vi "Win Host - Decimate Image Low Level.vi"(8 "error in (no error)":errorcluster, 11 "Image Path":path) -> (0 "error out":errorcluster, 1 "ImageData":T1, 2 "Rectangle":T2, 3 "new picture":picture)   [LabVIEW 2024]
uses:
  <vilib>/picture/picture.llb/imagedata.ctl
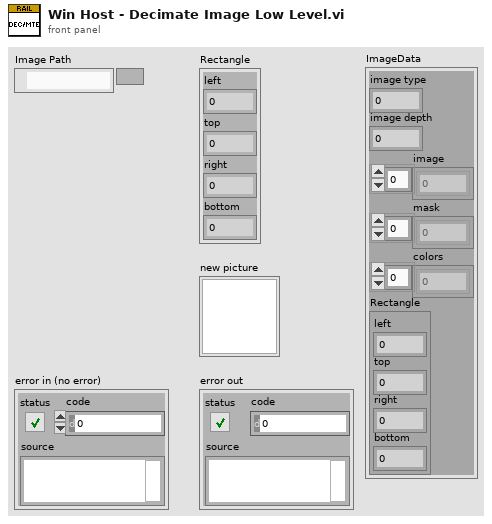
[diagram p1: front panel]
types:
  T1 = typedef "imagedata.ctl" = cluster{"image type":i32, "image depth":i32, "image":u8[], "mask":u8[], "colors":u32[], "Rectangle":cluster{"left":i16, "top":i16, "right":i16, "bottom":i16}}
  T2 = cluster{"left":i16, "top":i16, "right":i16, "bottom":i16}
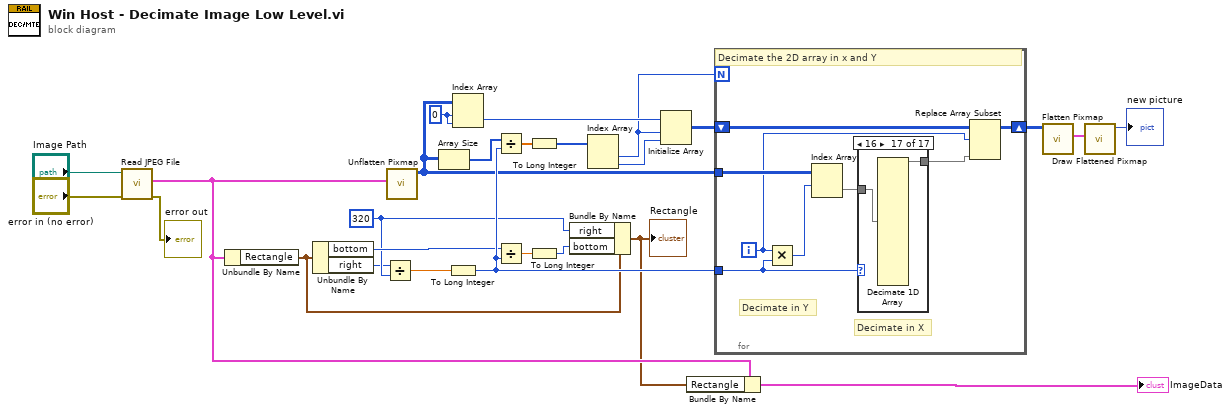
[diagram p0: block diagram]
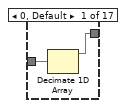
[diagram p2: hidden frame]
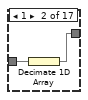
[diagram p3: hidden frame]
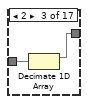
[diagram p4: hidden frame]
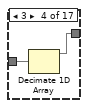
[diagram p5: hidden frame]
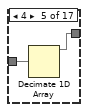
[diagram p6: hidden frame]
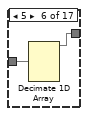
[diagram p7: hidden frame]
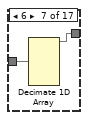
[diagram p8: hidden frame]
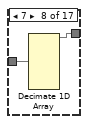
[diagram p9: hidden frame]
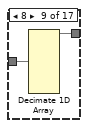
[diagram p10: hidden frame]
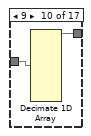
[diagram p11: hidden frame]
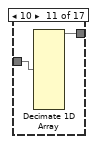
[diagram p12: hidden frame]
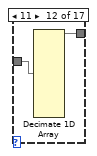
[diagram p13: hidden frame]
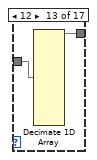
[diagram p14: hidden frame]
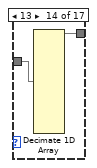
[diagram p15: hidden frame]
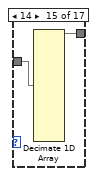
[diagram p16: hidden frame]
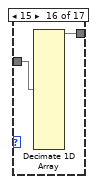
[diagram p17: hidden frame]
diagram:
  w10 = 0 ("disabled index (col)")
  w22 = i16 320 ("y")
  n1 = call <vilib>:"Read JPEG File.vi"("error in (no error)"="error in (no error)", "path to JPEG file"="Image Path") -> ("error out"=→"error out":errorcluster, "image data"=w3:T1)  [unwired: 7 in, 1 out]
  n2 = Unbundle By Name(w3) -> ("Rectangle"=w21:T2)
  n3 = Unbundle By Name(w21) -> ("bottom"=w24:i16, "right"=w19:i16)
  n4 = Divide(x=w19, y=w22) -> (x/y=w16:dbl)
  n5 = call <vilib>:"Unflatten Pixmap.vi"("image data"=w3) -> ("24-bit pixmap"=w9:u32[][])  [unwired: 4 in, 6 out]
  n6 = Array Size(array=w9) -> (size(s)=w15:i32[])
  n7 = To Long Integer(number=w16) -> (32bit integer=w25:i32)
  n8 = Index Array(array=w9, index (row)=w10, index (col)=w10) -> (element=w11:u32)
  n9 = Divide(x=w15, y=w25) -> (x/y=w17:dbl[])
  n10 = Divide(x=w24, y=w25) -> (x/y=w23:dbl)
  n11 = To Long Integer(number=w17) -> (32bit integer=w18:i32[])
  n12 = To Long Integer(number=w23) -> (32bit integer=w26:i32)
  n13 = Bundle By Name(cluster=w21, "right"=w22, "bottom"=w26) -> (w2:T2)
  "Rectangle" <- w2
  n14 = Index Array(array=w18) -> (element #1=w8:i32, element #2=w7:i32)  [unwired: 2 in]
  n15 = Initialize Array(w11, w8, w7) -> (w6:u32[][])
  n16 = Bundle By Name(cluster=w3, "Rectangle"=w2) -> (→"ImageData":T1)
  n17 = for {
    N: w8 -> [_]
    shift-right: [w34] -> w12
    shift-left: w6 -> [w33]
    tunnel: w9 -> [w32]
    tunnel: w25 -> [w27]
    i -> [w29]
    # "Decimate in X"
    # "Decimate in Y"
    # "Decimate the 2D array in x and Y"
    n18 = Multiply(x=w29, y=w27) -> (x*y=w28:i32)
    n19 = Index Array(array=w32, index (row)=w28) -> (element=w31:u32[])  [unwired: 1 in]
    n20 = case shown="16" w27 {
      tunnel: w31 -> [w36 w38 w40 w42 w44 w46 w48 w50 w52 w54 w56 w58 w60 w62 w64 w66 w68]
      tunnel: [w35 w37 w39 w41 w43 w45 w47 w49 w51 w53 w55 w57 w59 w61 w63 w65 w67] -> w30
      frame 0, Default {
        n21 = Decimate 1D Array(w36) -> (w35:u32[])  [unwired: 2 out]
      }
      frame 1 {
        n22 = Decimate 1D Array(w38) -> (w37:u32[])
      }
      frame 2 {
        n23 = Decimate 1D Array(w40) -> (w39:u32[])  [unwired: 1 out]
      }
      frame 3 {
        n24 = Decimate 1D Array(w42) -> (w41:u32[])  [unwired: 2 out]
      }
      frame 4 {
        n25 = Decimate 1D Array(w44) -> (w43:u32[])  [unwired: 3 out]
      }
      frame 5 {
        n26 = Decimate 1D Array(w46) -> (w45:u32[])  [unwired: 4 out]
      }
      frame 6 {
        n27 = Decimate 1D Array(w48) -> (w47:u32[])  [unwired: 5 out]
      }
      frame 7 {
        n28 = Decimate 1D Array(w50) -> (w49:u32[])  [unwired: 6 out]
      }
      frame 8 {
        n29 = Decimate 1D Array(w52) -> (w51:u32[])  [unwired: 7 out]
      }
      frame 9 {
        n30 = Decimate 1D Array(w54) -> (w53:u32[])  [unwired: 8 out]
      }
      frame 10 {
        n31 = Decimate 1D Array(w56) -> (w55:u32[])  [unwired: 9 out]
      }
      frame 11 {
        n32 = Decimate 1D Array(w58) -> (w57:u32[])  [unwired: 10 out]
      }
      frame 12 {
        n33 = Decimate 1D Array(w60) -> (w59:u32[])  [unwired: 11 out]
      }
      frame 13 {
        n34 = Decimate 1D Array(w62) -> (w61:u32[])  [unwired: 12 out]
      }
      frame 14 {
        n35 = Decimate 1D Array(w64) -> (w63:u32[])  [unwired: 13 out]
      }
      frame 15 {
        n36 = Decimate 1D Array(w66) -> (w65:u32[])  [unwired: 14 out]
      }
      frame 16 {
        n37 = Decimate 1D Array(w68) -> (w67:u32[])  [unwired: 15 out]
      }
    }
    n38 = Replace Array Subset(array=w33, new element=w30, index (row)=w29) -> (w34:u32[][])  [unwired: 1 in]
  }
  n39 = call <vilib>:"Flatten Pixmap.vi"("24-bit pixmap"=w12) -> ("image data"=w13:T1)  [unwired: 10 in]
  n40 = call <vilib>:"Draw Flattened Pixmap.vi"("image data"=w13) -> ("new picture"=→"new picture":picture)  [unwired: 8 in]
